vi "S706 Statusword.vi"() -> ()   [LabVIEW 2014]
uses:
  <vilib>/CANopenLib/CANOPEN.llb/CANopen SDO Create.vi
  <vilib>/CANopenLib/CANOPEN.llb/CANopen Interface Close.vi
panel:
  out "13 Referenzfahrtfehler":bool
  out "12 Referenzfahrt durchgeführt":bool
  out "11 internal_limit_active":bool
  out "10 target_reached":bool
  out "9 remote (kann kommunizieren)":bool
  out "8":bool
  out "7 warning":bool
  out "6 switch on disable":bool
  out "5 quick stop":bool
  out "4 voltage enabled":bool
  out "3 fault":bool
  out "2 operation enable":bool
  out "1 switched on":bool
  out "0 ready to switch on":bool
  out "error out":errorcluster
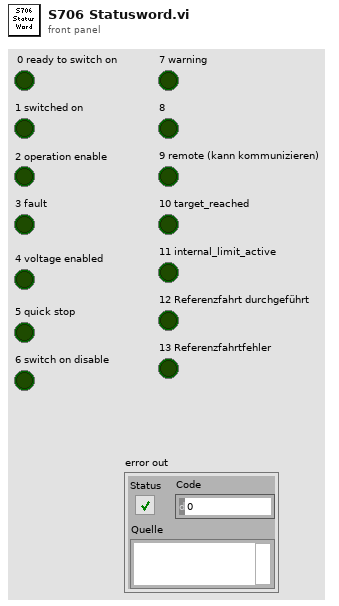
[diagram p1: front panel]
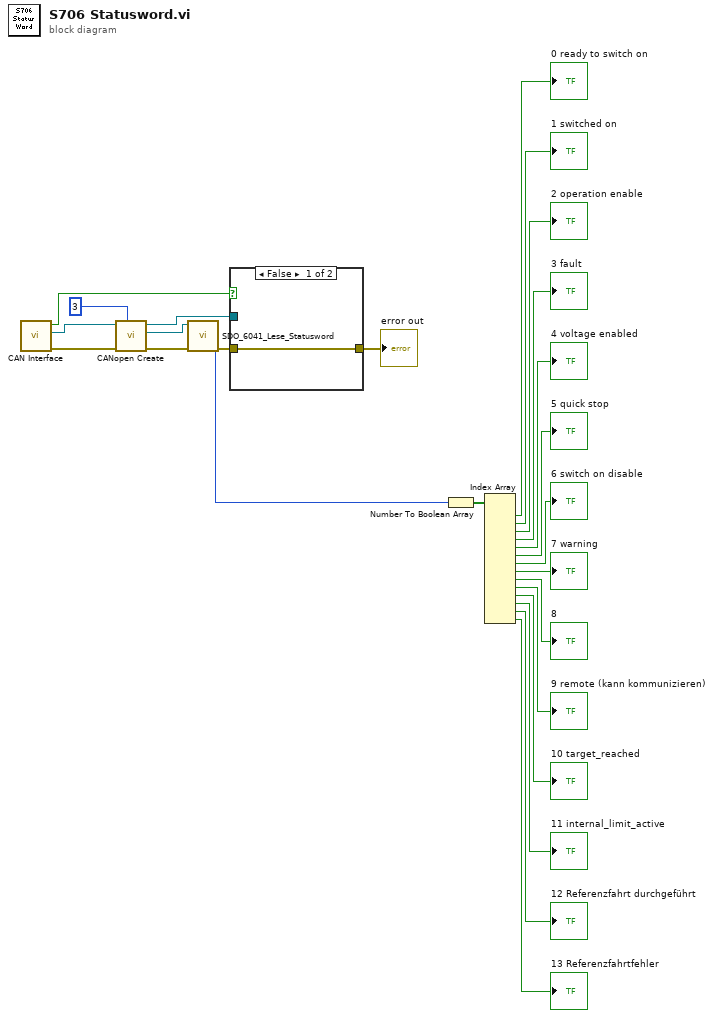
[diagram p0: block diagram]
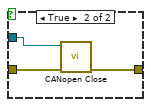
[diagram p2: hidden frame]
diagram:
  n1 = call "CAN Interface.vi"() -> ("error out"=w20:errorcluster, "interface object out"=w19:refnum<k20>, "Interface schließen?"=w18:bool)  [unwired: 9 in]
  n2 = call-poly <vilib>:"CANopen Create.vi"("node-ID"=u8 3, "error in (no error)"=w20, "interface object in"=w19) -> ("error out"=w22:errorcluster, "SDO object out"=w24:refnum<k20>, "interface object out"=w23:refnum<k20>)  [unwired: 6 in]
  n3 = call "SDO_6041_Lese_Statusword.vi"("error in (no error)"=w22, "SDO object in"=w24) -> ("error out"=w21:errorcluster, "U16 data"=w1:u16)  [unwired: 6 in, 2 out]
  n4 = case shown="False" w18 {
    tunnel: w23 -> [_ w29]
    tunnel: w21 -> [w26 w28]
    tunnel: [w26 w27] -> w25
    frame False {
    }
    frame True {
      n5 = call-poly <vilib>:"CANopen Close.vi"("error in (no error)"=w28, "interface object in"=w29) -> ("error out"=w27:errorcluster)  [unwired: 9 in]
    }
  }
  "error out" <- w25
  n6 = Number To Boolean Array(number=w1) -> (Boolean array=w16:bool[])
  n7 = Index Array(array=w16) -> (element #1=→"0 ready to switch on":bool, element #2=→"1 switched on":bool, element #3=→"2 operation enable":bool, element #4=→"3 fault":bool, element #5=→"4 voltage enabled":bool, element #6=→"5 quick stop":bool, element #7=→"6 switch on disable":bool, element #8=→"7 warning":bool, element #9=→"8":bool, element #10=→"9 remote (kann kommunizieren)":bool, element #11=→"10 target_reached":bool, element #12=→"11 internal_limit_active":bool, element #13=→"12 Referenzfahrt durchgeführt":bool, element #14=→"13 Referenzfahrtfehler":bool)  [unwired: 14 in]
